vi "open_tilt_stage_motor.vi"(4 "error in (no error)":errorcluster, 6 "Open device?":bool, 7 "DeviceKey In":string) -> (0 "error out":errorcluster, 1 "CmdLib Out":refnum<k24>, 2 "Device Address":i32, 3 "DeviceKey Out":string)   [LabVIEW 2016]
uses:
  C:/Users/UsphereLab/Documents/GitHub/Optlev/LabView Code/Examples/Tilt Stage/CmdLib.dll
  Examples/Tilt Stage/CmdLib.dll
panel:
  out "DeviceKey Out 0":string
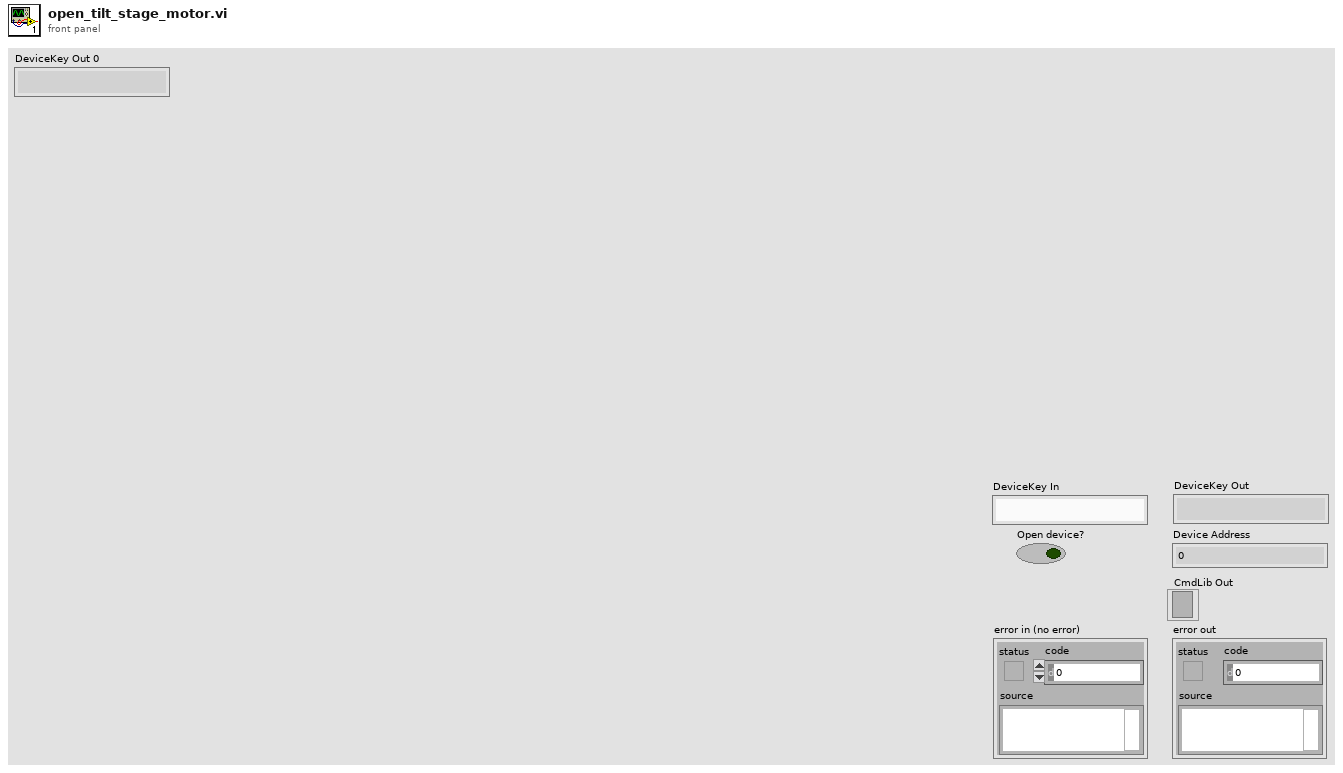
[diagram p1: front panel]
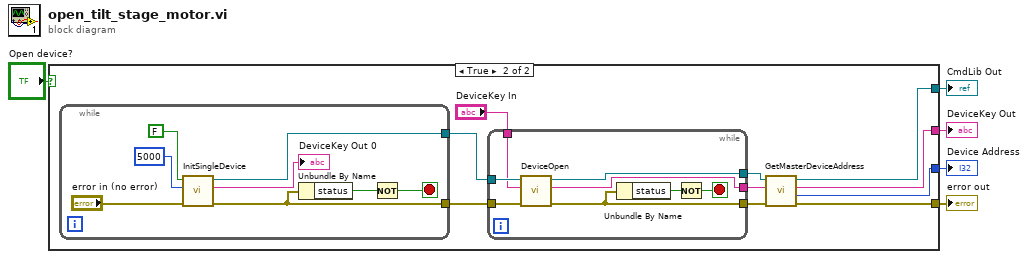
[diagram p0: block diagram]
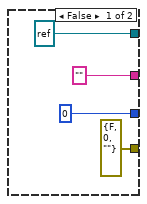
[diagram p2: hidden frame]
diagram:
  n1 = case shown="True" "Open device?" {
    tunnel: [errorcluster {"status"=FALSE, "code"=0, "source"=""} ("error out") w13] -> w4
    tunnel: [0 ("Device Address") w12] -> w3
    tunnel: ["" ("DeviceKey Out") w11] -> w2
    tunnel: [refnum<k24> refnum ("CmdLib Out") w10] -> w1
    frame False {
    }
    frame True {
      n2 = while {
        tunnel: [w25] -> w19
        tunnel: [w23] -> w18
        stop <- w21 stop-if-true
        n3 = call "InitSingleDevice.vi"("error in (no error)"="error in (no error)", "msecDelayForDiscovery"=5000, "logging"=FALSE) -> ("error out"=w23:errorcluster, "DeviceKey Out"=→"DeviceKey Out 0":string, "CmdLib Out"=w25:refnum<k24>)  [unwired: 2 in]
        n4 = Unbundle By Name(w23) -> ("status"=w22:bool)
        n5 = Not(x=w22) -> (.not. x?=w21:bool)
      }
      n6 = while {
        tunnel: w19 -> [w35]
        tunnel: [w32] -> w16
        tunnel: "DeviceKey In" -> [w31]
        tunnel: [w33] -> w17
        tunnel: w18 -> [w34]
        tunnel: [w30] -> w14
        stop <- w28 stop-if-true
        n7 = call "DeviceOpen.vi"("error in (no error)"=w34, "DeviceKey In"=w31, "CmdLib In"=w35) -> ("error out"=w30:errorcluster, "DeviceKey Out"=w33:string, "CmdLib Out"=w32:refnum<k24>)  [unwired: 2 in]
        n8 = Unbundle By Name(w30) -> ("status"=w29:bool)
        n9 = Not(x=w29) -> (.not. x?=w28:bool)
      }
      n10 = call "GetMasterDeviceAddress.vi"("error in (no error)"=w14, "DeviceKey In"=w17, "CmdLib In"=w16) -> ("error out"=w13:errorcluster, "Device Address"=w12:i32, "DeviceKey Out"=w11:string, "CmdLib Out"=w10:refnum<k24>)  [unwired: 1 in]
    }
  }
  "error out" <- w4
  "Device Address" <- w3
  "DeviceKey Out" <- w2
  "CmdLib Out" <- w1
